vi "rsidr_core_global.vi"() -> ()   [LabVIEW 2020, in "Rohde&Schwarz RTx Oscilloscopes.lvlib"] (continued)
{"Level"=2, "Class Only"=TRUE, "Identifier"="", "Descriptive Name"="ARINC 429", "Data Type"=0, "Command"="", "Access"=0, "Range Table"="", "Read Callback"="", "Write Callback"="", "Supported Models"="", "Instrument Options"="", "Flags"=0, "Help"="ARINC 429 (Option K7)"}, {"Level"=3, "Class Only"=FALSE, "Identifier"="RSRTX_ATTR_PROTOCOL_ARINC429_SOURCE", "Descriptive Name"="Protocol ARINC429 Source", "Data Type"=0, "Command"="BUS{SerialBus}:ARINc:SOUR", "Access"=2, "Range Table"="rsrtx_rngSource", "Read Callback"="", "Write Callback"="", "Supported Models"="RTM|RTA", "Instrument Options"="", "Flags"=0, "Help"="Sets the channel for the signal source.\n\nAvailable Repeated Capabilities:\nSerialBus: SB1, SB2, SB3, SB4\r\n\nRemote-control command(s):\nBUS<b>:ARINc:SOURce"}, {"Level"=3, "Class Only"=FALSE, "Identifier"="RSRTX_ATTR_PROTOCOL_ARINC429_POLARITY", "Descriptive Name"="Protocol ARINC429 Polarity", "Data Type"=0, "Command"="BUS{SerialBus}:ARIN:POL", "Access"=2, "Range Table"="rsrtx_rngProtocolARINC429Polarity", "Read Callback"="", "Write Callback"="", "Supported Models"="RTM|RTA", "Instrument Options"="", "Flags"=0, "Help"="Sets the wire on which the bus signal is measured.\n\nAvailable Repeated Capabilities:\nSerialBus: SB1, SB2, SB3, SB4\r\n\nRemote-control command(s):\nBUS<b>:ARINc:POLarity"}, {"Level"=3, "Class Only"=FALSE, "Identifier"="RSRTX_ATTR_PROTOCOL_ARINC429_BIT_RATE_MODE", "Descriptive Name"="Protocol ARINC429 Bit Rate Mode", "Data Type"=0, "Command"="BUS{SerialBus}:ARIN:BRM", "Access"=2, "Range Table"="rsrtx_rngProtocolARINC429BitRateMode", "Read Callback"="", "Write Callback"="", "Supported Models"="RTM|RTA", "Instrument Options"="", "Flags"=0, "Help"="Sets the bit rate mode to high or low speed.\n\nAvailable Repeated Capabilities:\nSerialBus: SB1, SB2, SB3, SB4\r\n\nRemote-control command(s):\nBUS<b>:ARINc:BRMode"}, {"Level"=3, "Class Only"=FALSE, "Identifier"="RSRTX_ATTR_PROTOCOL_ARINC429_BIT_RATE", "Descriptive Name"="Protocol ARINC429 Bit Rate", "Data Type"=1, "Command"="BUS{SerialBus}:ARIN:BRV", "Access"=2, "Range Table"="", "Read Callback"="", "Write Callback"="", "Supported Models"="RTM|RTA", "Instrument Options"="", "Flags"=0, "Help"="Sets the number of transmitted bits per second.\n\nAvailable Repeated Capabilities:\nSerialBus: SB1, SB2, SB3, SB4\r\n\nRemote-control command(s):\nBUS<b>:ARINc:BRValue"}, {"Level"=3, "Class Only"=FALSE, "Identifier"="RSRTX_ATTR_PROTOCOL_ARINC429_THRESHOLD_HIGH", "Descriptive Name"="Protocol ARINC429 Threshold High", "Data Type"=1, "Command"="BUS{SerialBus}:ARIN:THR:HIGH", "Access"=2, "Range Table"="rsrtx_rngProtocolARINC429ThresholdHigh", "Read Callback"="", "Write Callback"="", "Supported Models"="RTM|RTA", "Instrument Options"="", "Flags"=0, "Help"="Sets the high threshold level of the signal.\n\nAvailable Repeated Capabilities:\nSerialBus: SB1, SB2, SB3, SB4\r\n\nRemote-control command(s):\nBUS<b>:ARINc:THReshold:HIGH"}, {"Level"=3, "Class Only"=FALSE, "Identifier"="RSRTX_ATTR_PROTOCOL_ARINC429_THRESHOLD_LOW", "Descriptive Name"="Protocol ARINC429 Threshold Low", "Data Type"=1, "Command"="BUS{SerialBus}:ARIN:THR:LOW", "Access"=2, "Range Table"="rsrtx_rngProtocolARINC429ThresholdLow", "Read Callback"="", "Write Callback"="", "Supported Models"="RTM|RTA", "Instrument Options"="", "Flags"=0, "Help"="Sets the low threshold level of the signal.\n\nAvailable Repeated Capabilities:\nSerialBus: SB1, SB2, SB3, SB4\r\n\nRemote-control command(s):\nBUS<b>:ARINc:THReshold:LOW"}, {"Level"=3, "Class Only"=FALSE, "Identifier"="RSRTX_ATTR_PROTOCOL_ARINC429_DATA_FORMAT", "Descriptive Name"="Protocol ARINC429 Data Format", "Data Type"=0, "Command"="BUS{SerialBus}:ARIN:DATA:FORM", "Access"=2, "Range Table"="rsrtx_rngProtocolARINC429DataFormat", "Read Callback"="", "Write Callback"="", "Supported Models"="RTM|RTA", "Instrument Options"="", "Flags"=0, "Help"="Sets the decoding data format for the specified ARINC 429 bus.\n\nAvailable Repeated Capabilities:\nSerialBus: SB1, SB2, SB3, SB4\r\n\nRemote-control command(s):\nBUS<b>:ARINc:DATA:FORMat"}, {"Level"=3, "Class Only"=TRUE, "Identifier"="", "Descriptive Name"="Decoding Results", "Data Type"=0, "Command"="", "Access"=0, "Range Table"="", "Read Callback"="", "Write Callback"="", "Supported Models"="", "Instrument Options"="", "Flags"=0, "Help"="Returns the decoding result of the specified word."}, {"Level"=4, "Class Only"=FALSE, "Identifier"="RSRTX_ATTR_PROTOCOL_ARINC429_WORD_COUNT", "Descriptive Name"="Protocol ARINC429 Word Count", "Data Type"=0, "Command"="BUS{SerialBus}:ARIN:WCO?", "Access"=0, "Range Table"="", "Read Callback"="", "Write Callback"="", "Supported Models"="RTM|RTA", "Instrument Options"="", "Flags"=0, "Help"="Returns the number of decoded words.\n\nAvailable Repeated Capabilities:\nSerialBus: SB1, SB2, SB3, SB4\r\n\nRemote-control command(s):\nBUS<b>:ARINc:WCOunt?"}, {"Level"=4, "Class Only"=FALSE, "Identifier"="RSRTX_ATTR_PROTOCOL_ARINC429_SELECTED_WORD", "Descriptive Name"="Protocol ARINC429 Selected Word", "Data Type"=0, "Command"="", "Access"=2, "Range Table"="", "Read Callback"="", "Write Callback"="", "Supported Models"="", "Instrument Options"="", "Flags"=0, "Help"="Sets selector repeated capability Word.\n\nAvailable Repeated Capabilities:\nNone\n\nRemote-control command(s):\n"}, {"Level"=4, "Class Only"=FALSE, "Identifier"="RSRTX_ATTR_PROTOCOL_ARINC429_WORD_STATUS", "Descriptive Name"="Protocol ARINC429 Word Status", "Data Type"=0, "Command"="BUS{SerialBus}:ARIN:WORD<Word>:STAT?", "Access"=0, "Range Table"="rsrtx_rngARINC429WordStatus", "Read Callback"="rsrtx_FormatARINCWordRepCapInt_ReadCallback.vi", "Write Callback"="", "Supported Models"="RTM|RTA", "Instrument Options"="", "Flags"=0, "Help"="Returns the status of the specified word.\n\nAvailable Repeated Capabilities:\nSerialBus: SB1, SB2, SB3, SB4\r\n\nRemote-control command(s):\nBUS<b>:ARINc:WORD<n>:STATus?"}, {"Level"=4, "Class Only"=FALSE, "Identifier"="RSRTX_ATTR_PROTOCOL_ARINC429_WORD_START", "Descriptive Name"="Protocol ARINC429 Word Start", "Data Type"=1, "Command"="BUS{SerialBus}:ARIN:WORD<Word>:STAR?", "Access"=0, "Range Table"="", "Read Callback"="rsrtx_FormatARINCWordRepCapReal_ReadCallback.vi", "Write Callback"="", "Supported Models"="RTM|RTA", "Instrument Options"="", "Flags"=0, "Help"="Returns the start time of the specified word.\n\nAvailable Repeated Capabilities:\nSerialBus: SB1, SB2, SB3, SB4\r\n\nRemote-control command(s):\nBUS<b>:ARINc:WORD<n>:STARt?"}, {"Level"=4, "Class Only"=FALSE, "Identifier"="RSRTX_ATTR_PROTOCOL_ARINC429_WORD_STOP", "Descriptive Name"="Protocol ARINC429 Word Stop", "Data Type"=1, "Command"="BUS{SerialBus}:ARIN:WORD<Word>:STOP?", "Access"=0, "Range Table"="", "Read Callback"="rsrtx_FormatARINCWordRepCapReal_ReadCallback.vi", "Write Callback"="", "Supported Models"="RTM|RTA", "Instrument Options"="", "Flags"=0, "Help"="Returns the start time of the specified word.\n\nAvailable Repeated Capabilities:\nSerialBus: SB1, SB2, SB3, SB4\r\n\nRemote-control command(s):\nBUS<b>:ARINc:WORD<n>:STOP?"}, {"Level"=4, "Class Only"=FALSE, "Identifier"="RSRTX_ATTR_PROTOCOL_ARINC429_WORD_SDI", "Descriptive Name"="Protocol ARINC429 Word SDI", "Data Type"=0, "Command"="BUS{SerialBus}:ARIN:WORD<Word>:SDI?", "Access"=0, "Range Table"="", "Read Callback"="rsrtx_FormatARINCWordRepCapInt_ReadCallback.vi", "Write Callback"="", "Supported Models"="RTM|RTA", "Instrument Options"="", "Flags"=0, "Help"="Returns the source/destination identifier (SDI) bits of the specified word.\n\nAvailable Repeated Capabilities:\nSerialBus: SB1, SB2, SB3, SB4\r\n\nRemote-control command(s):\nBUS<b>:ARINc:WORD<n>:SDI?"}, {"Level"=4, "Class Only"=FALSE, "Identifier"="RSRTX_ATTR_PROTOCOL_ARINC429_WORD_SSM", "Descriptive Name"="Protocol ARINC429 Word SSM", "Data Type"=0, "Command"="BUS{SerialBus}:ARIN:WORD<Word>:SSM?", "Access"=0, "Range Table"="", "Read Callback"="rsrtx_FormatARINCWordRepCapInt_ReadCallback.vi", "Write Callback"="", "Supported Models"="RTM|RTA", "Instrument Options"="", "Flags"=0, "Help"="Returns the source/destination identifier (SDI) bits of the specified word.\n\nAvailable Repeated Capabilities:\nSerialBus: SB1, SB2, SB3, SB4\r\n\nRemote-control command(s):\nBUS<b>:ARINc:WORD<n>:SSM?"}, {"Level"=4, "Class Only"=FALSE, "Identifier"="RSRTX_ATTR_PROTOCOL_ARINC429_WORD_LABEL", "Descriptive Name"="Protocol ARINC429 Word Label", "Data Type"=2, "Command"="BUS{SerialBus}:ARIN:WORD<Word>:LAB?", "Access"=0, "Range Table"="", "Read Callback"="rsrtx_FormatARINCWordRepCapString_ReadCallback.vi", "Write Callback"="", "Supported Models"="RTM|RTA", "Instrument Options"="", "Flags"=0, "Help"="Returns the label of the specified word.\n\nAvailable Repeated Capabilities:\nSerialBus: SB1, SB2, SB3, SB4\r\n\nRemote-control command(s):\nBUS<b>:ARINc:WORD<n>:LABel?"}, {"Level"=4, "Class Only"=FALSE, "Identifier"="RSRTX_ATTR_PROTOCOL_ARINC429_WORD_LABEL_VALUE", "Descriptive Name"="Protocol ARINC429 Word Label Value", "Data Type"=0, "Command"="BUS{SerialBus}:ARIN:WORD<Word>:LAB:VAL?", "Access"=0, "Range Table"="", "Read Callback"="rsrtx_FormatARINCWordRepCapInt_ReadCallback.vi", "Write Callback"="", "Supported Models"="RTM|RTA", "Instrument Options"="", "Flags"=0, "Help"="Returns the decimal value of the label of the specified word.\n\nAvailable Repeated Capabilities:\nSerialBus: SB1, SB2, SB3, SB4\r\n\nRemote-control command(s):\nBUS<b>:ARINc:WORD<n>:LABel[:VALue]?"}, {"Level"=4, "Class Only"=FALSE, "Identifier"="RSRTX_ATTR_PROTOCOL_ARINC429_WORD_PATTERN", "Descriptive Name"="Protocol ARINC429 Word Pattern", "Data Type"=0, "Command"="BUS{SerialBus}:ARIN:WORD<Word>:PATT?", "Access"=0, "Range Table"="", "Read Callback"="rsrtx_FormatARINCWordRepCapInt_ReadCallback.vi", "Write Callback"="", "Supported Models"="RTM|RTA", "Instrument Options"="", "Flags"=0, "Help"="Returns all 32 bits of a data word as decimal value.\n\nAvailable Repeated Capabilities:\nSerialBus: SB1, SB2, SB3, SB4\r\n\nRemote-control command(s):\nBUS<b>:ARINc:WORD<n>:PATTern?"}, {"Level"=4, "Class Only"=FALSE, "Identifier"="RSRTX_ATTR_PROTOCOL_ARINC429_WORD_PARITY", "Descriptive Name"="Protocol ARINC429 Word Parity", "Data Type"=0, "Command"="BUS{SerialBus}:ARIN:WORD<Word>:PAR?", "Access"=0, "Range Table"="", "Read Callback"="rsrtx_FormatARINCWordRepCapInt_ReadCallback.vi", "Write Callback"="", "Supported Models"="RTM|RTA", "Instrument Options"="", "Flags"=0, "Help"="Returns the parity of the specified word.\n\nAvailable Repeated Capabilities:\nSerialBus: SB1, SB2, SB3, SB4\r\n\nRemote-control command(s):\nBUS<b>:ARINc:WORD<n>:PARity?"}, {"Level"=4, "Class Only"=FALSE, "Identifier"="RSRTX_ATTR_PROTOCOL_ARINC429_WORD_FORMAT", "Descriptive Name"="Protocol ARINC429 Word Format", "Data Type"=0, "Command"="BUS{SerialBus}:ARIN:WORD<Word>:FORM?", "Access"=0, "Range Table"="rsrtx_rngProtocolARINC429DataFormat", "Read Callback"="rsrtx_FormatARINCWordRepCapInt_ReadCallback.vi", "Write Callback"="", "Supported Models"="RTM|RTA", "Instrument Options"="", "Flags"=0, "Help"="Returns the format of the sepcified word.\n\nAvailable Repeated Capabilities:\nSerialBus: SB1, SB2, SB3, SB4\r\n\nRemote-control command(s):\nBUS<b>:ARINc:WORD<n>:FORMat?"}, {"Level"=4, "Class Only"=FALSE, "Identifier"="RSRTX_ATTR_PROTOCOL_ARINC429_WORD_DATA", "Descriptive Name"="Protocol ARINC429 Word Data", "Data Type"=0, "Command"="BUS{SerialBus}:ARIN:WORD<Word>:DATA:VAL?", "Access"=0, "Range Table"="", "Read Callback"="rsrtx_FormatARINCWordRepCapInt_ReadCallback.vi", "Write Callback"="", "Supported Models"="", "Instrument Options"="", "Flags"=0, "Help"="Returns the decimal value of the data of the specified word.\n\nAvailable Repeated Capabilities:\nSerialBus: SB1, SB2, SB3, SB4\r\n\nRemote-control command(s):\nBUS<b>:ARINc:WORD<n>:DATA[:VALue]?"}, {"Level"=1, "Class Only"=TRUE, "Identifier"="", "Descriptive Name"="Power Analysis", "Data Type"=0, "Command"="", "Access"=0, "Range Table"="", "Read Callback"="", "Write Callback"="", "Supported Models"="", "Instrument Options"="", "Flags"=0, "Help"="Power Analysis."}, {"Level"=2, "Class Only"=FALSE, "Identifier"="RSRTX_ATTR_POWER_ANALYSIS_ENABLED", "Descriptive Name"="Power Analysis Enabled", "Data Type"=3, "Command"="POW:ENAB", "Access"=2, "Range Table"="", "Read Callback"="", "Write Callback"="", "Supported Models"="RTM|RTA", "Instrument Options"="", "Flags"=0, "Help"="Enables the power analysis.\n\nAvailable Repeated Capabilities:\nNone\n\nRemote-control command(s):\nPOWer:ENABle"}, {"Level"=2, "Class Only"=FALSE, "Identifier"="RSRTX_ATTR_POWER_ANALYSIS_TYPE", "Descriptive Name"="Power Analysis Type", "Data Type"=0, "Command"="POW:ATYP", "Access"=2, "Range Table"="rsrtx_rngPowerAnalysisType", "Read Callback"="", "Write Callback"="", "Supported Models"="RTM|RTA", "Instrument Options"="", "Flags"=0, "Help"="Selects power analysis type.\n\nAvailable Repeated Capabilities:\nNone\n\nRemote-control command(s):\nPOWer:ATYPe"}, {"Level"=2, "Class Only"=FALSE, "Identifier"="RSRTX_ATTR_POWER_ANALYSIS_RESULT_TABLE_ENABLED", "Descriptive Name"="Power Analysis Result Table Enabled", "Data Type"=3, "Command"="POW:RES:TABL", "Access"=2, "Range Table"="", "Read Callback"="", "Write Callback"="", "Supported Models"="RTM|RTA", "Instrument Options"="", "Flags"=0, "Help"="Displays or hides the result table. Available for harmonic and spectrum power measurements.\n\nAvailable Repeated Capabilities:\nNone\n\nRemote-control command(s):\nPOWer:RESult:TABLe"}, {"Level"=2, "Class Only"=FALSE, "Identifier"="RSRTX_ATTR_POWER_ANALYSIS_RESET_STATISTICS", "Descriptive Name"="Power Analysis Reset Statistics", "Data Type"=4, "Command"="POW:STAT:RES", "Access"=1, "Range Table"="", "Read Callback"="", "Write Callback"="", "Supported Models"="RTM|RTA", "Instrument Options"="", "Flags"=0, "Help"="Resets statistics.\n\nAvailable Repeated Capabilities:\nNone\n\nRemote-control command(s):\nPOWer:STATistics:RESet"}, {"Level"=2, "Class Only"=FALSE, "Identifier"="RSRTX_ATTR_POWER_ANALYSIS_STATISTICS_VISIBLE", "Descriptive Name"="Power Analysis Statistics Visible", "Data Type"=3, "Command"="POW:STAT:VIS", "Access"=2, "Range Table"="", "Read Callback"="", "Write Callback"="", "Supported Models"="RTM|RTA", "Instrument Options"="", "Flags"=0, "Help"="Visible statistics\n\nAvailable Repeated Capabilities:\nNone\n\nRemote-control command(s):\nPOWer:STATistics:VISible"}, {"Level"=2, "Class Only"=FALSE, "Identifier"="RSRTX_ATTR_POWER_ANALYSIS_START_DESKEW", "Descriptive Name"="Power Analysis Start Deskew", "Data Type"=4, "Command"="POW:DESK", "Access"=1, "Range Table"="", "Read Callback"="", "Write Callback"="", "Supported Models"="RTM|RTA", "Instrument Options"="", "Flags"=1, "Help"="Starts the automatic deskew procedure to align the waveforms of all visible channels. It is necessary to deskew if a current and a voltage probe is used in the measurment. Use the R&S RT-ZF20 power deskew fixture to deskew the probes.\n\nAvailable Repeated Capabilities:\nNone\n\nRemote-control command(s):\nPOWer:DESKew[:EXECute]"}, {"Level"=2, "Class Only"=FALSE, "Identifier"="RSRTX_ATTR_POWER_ANALYSIS_ZERO_OFFSET", "Descriptive Name"="Power Analysis Zero Offset", "Data Type"=4, "Command"="POW:ZOFF", "Access"=1, "Range Table"="", "Read Callback"="", "Write Callback"="", "Supported Models"="RTM|RTA", "Instrument Options"="", "Flags"=1, "Help"="Sets zero offset.\n\nAvailable Repeated Capabilities:\nNone\n\nRemote-control command(s):\nPOWer:ZOFFset[:EXECute]"}, {"Level"=2, "Class Only"=FALSE, "Identifier"="RSRTX_ATTR_POWER_ANALYSIS_AUTOSET", "Descriptive Name"="Power Analysis Autoset", "Data Type"=4, "Command"="POW:AUT", "Access"=1, "Range Table"="", "Read Callback"="", "Write Callback"="", "Supported Models"="RTM|RTA", "Instrument Options"="", "Flags"=0, "Help"="Starts power analysis autoset.\n\nAvailable Repeated Capabilities:\nNone\n\nRemote-control command(s):\nPOWer:AUToscale"}, {"Level"=2, "Class Only"=FALSE, "Identifier"="RSRTX_ATTR_POWER_ANALYSIS_AUTOSET_CURRENT", "Descriptive Name"="Power Analysis Autoset Current", "Data Type"=4, "Command"="POW:AUT:CURR", "Access"=1, "Range Table"="", "Read Callback"="", "Write Callback"="", "Supported Models"="RTM|RTA", "Instrument Options"="", "Flags"=0, "Help"="Starts power analysis current autoset.\n\nAvailable Repeated Capabilities:\nNone\n\nRemote-control command(s):\nPOWer:AUToscale:CURRent"}, {"Level"=2, "Class Only"=FALSE, "Identifier"="RSRTX_ATTR_POWER_ANALYSIS_AUTOSET_VOLTAGE", "Descriptive Name"="Power Analysis Autoset Voltage", "Data Type"=4, "Command"="POW:AUT:VOLT", "Access"=1, "Range Table"="", "Read Callback"="", "Write Callback"="", "Supported Models"="RTM|RTA", "Instrument Options"="", "Flags"=0, "Help"="Starts power analysis voltage autoset.\n\nAvailable Repeated Capabilities:\nNone\n\nRemote-control command(s):\nPOWer:AUToscale:VOLTage"}, {"Level"=2, "Class Only"=TRUE, "Identifier"="", "Descriptive Name"="Source", "Data Type"=0, "Command"="", "Access"=0, "Range Table"="", "Read Callback"="", "Write Callback"="", "Supported Models"="", "Instrument Options"="", "Flags"=0, "Help"="Clas for attributes with Source repcap."}, {"Level"=3, "Class Only"=FALSE, "Identifier"="RSRTX_ATTR_POWER_ANALYSIS_VOLTAGE_SOURCE", "Descriptive Name"="Power Analysis Voltage Source", "Data Type"=0, "Command"="POW:SOUR:VOLT{SourceNumber}", "Access"=2, "Range Table"="rsrtx_rngPowerAnalysisSource", "Read Callback"="", "Write Callback"="", "Supported Models"="RTM|RTA", "Instrument Options"="", "Flags"=0, "Help"="Sets the channel for the voltage source input.\n\nAvailable Repeated Capabilities:\nSourceNumber: S1, S2, S3, S4\r\n\nRemote-control command(s):\nPOWer:SOURce:VOLTage<n>"}, {"Level"=3, "Class Only"=FALSE, "Identifier"="RSRTX_ATTR_POWER_ANALYSIS_CURRENT_SOURCE", "Descriptive Name"="Power Analysis Current Source", "Data Type"=0, "Command"="POW:SOUR:CURR{SourceNumber}", "Access"=2, "Range Table"="rsrtx_rngPowerAnalysisSource", "Read Callback"="", "Write Callback"="", "Supported Models"="RTM|RTA", "Instrument Options"="", "Flags"=0, "Help"="Sets the channel for the current source input.\n\nAvailable Repeated Capabilities:\nSourceNumber: S1, S2, S3, S4\r\n\nRemote-control command(s):\nPOWer:SOURce:CURRent<n>"}, {"Level"=2, "Class Only"=TRUE, "Identifier"="", "Descriptive Name"="Report", "Data Type"=0, "Command"="", "Access"=0, "Range Table"="", "Read Callback"="", "Write Callback"="", "Supported Models"="", "Instrument Options"="", "Flags"=0, "Help"="Power analysis report."}, {"Level"=3, "Class Only"=FALSE, "Identifier"="RSRTX_ATTR_POWER_ANALYSIS_ADD_REPORT", "Descriptive Name"="Power Analysis Add Report", "Data Type"=4, "Command"="POW:REP:ADD", "Access"=1, "Range Table"="", "Read Callback"="", "Write Callback"="", "Supported Models"="RTM|RTA", "Instrument Options"="", "Flags"=0, "Help"="Adds a power report.\n\nAvailable Repeated Capabilities:\nNone\n\nRemote-control command(s):\nPOWer:REPort:ADD"}, {"Level"=3, "Class Only"=FALSE, "Identifier"="RSRTX_ATTR_POWER_ANALYSIS_REPORT_DUT", "Descriptive Name"="Power Analysis Report DUT", "Data Type"=2, "Command"="POW:REP:DUT", "Access"=2, "Range Table"="", "Read Callback"="", "Write Callback"="", "Supported Models"="RTM|RTA", "Instrument Options"="", "Flags"=0, "Help"="Sets a device under test (DUT) value that can be shown at the titel page of a report.\n\nAvailable Repeated Capabilities:\nNone\n\nRemote-control command(s):\nPOWer:REPort:DUT"}, {"Level"=3, "Class Only"=FALSE, "Identifier"="RSRTX_ATTR_POWER_ANALYSIS_REPORT_USER", "Descriptive Name"="Power Analysis Report User", "Data Type"=2, "Command"="POW:REP:USER", "Access"=2, "Range Table"="", "Read Callback"="", "Write Callback"="", "Supported Models"="RTM|RTA", "Instrument Options"="", "Flags"=0, "Help"="Sets a user value that can be shown at the titel page of a report.\n\nAvailable Repeated Capabilities:\nNone\n\nRemote-control command(s):\nPOWer:REPort:USER"}, {"Level"=3, "Class Only"=FALSE, "Identifier"="RSRTX_ATTR_POWER_ANALYSIS_REPORT_SITE", "Descriptive Name"="Power Analysis Report Site", "Data Type"=2, "Command"="POW:REP:SITE", "Access"=2, "Range Table"="", "Read Callback"="", "Write Callback"="", "Supported Models"="RTM|RTA", "Instrument Options"="", "Flags"=0, "Help"="Sets a site value that can be shown at the titel page of a report.\n\nAvailable Repeated Capabilities:\nNone\n\nRemote-control command(s):\nPOWer:REPort:SITE"}, {"Level"=3, "Class Only"=FALSE, "Identifier"="RSRTX_ATTR_POWER_ANALYSIS_REPORT_TEMPERATURE", "Descriptive Name"="Power Analysis Report Temperature", "Data Type"=0, "Command"="POW:REP:TEMP", "Access"=2, "Range Table"="rsrtx_rngPowerAnalysisReportTemperature", "Read Callback"="", "Write Callback"="", "Supported Models"="RTM|RTA", "Instrument Options"="", "Flags"=0, "Help"="Sets a temperature value that can be shown at the titel page of a report.\n\nAvailable Repeated Capabilities:\nNone\n\nRemote-control command(s):\nPOWer:REPort:TEMPerature"}, {"Level"=3, "Class Only"=FALSE, "Identifier"="RSRTX_ATTR_POWER_ANALYSIS_REPORT_DESCRIPTION", "Descriptive Name"="Power Analysis Report Description", "Data Type"=2, "Command"="POW:REP:DESC", "Access"=2, "Range Table"="", "Read Callback"="", "Write Callback"="", "Supported Models"="RTM|RTA", "Instrument Options"="", "Flags"=0, "Help"="Sets a description that can be shown at the titel page of a report.\n\nAvailable Repeated Capabilities:\nNone\n\nRemote-control command(s):\nPOWer:REPort:DESCription"}, {"Level"=3, "Class Only"=FALSE, "Identifier"="RSRTX_ATTR_POWER_ANALYSIS_REPORT_OUTPUT_FOLDER", "Descriptive Name"="Power Analysis Report Output Folder", "Data Type"=2, "Command"="POW:REP:OUTP", "Access"=2, "Range Table"="", "Read Callback"="", "Write Callback"="", "Supported Models"="RTM|RTA", "Instrument Options"="", "Flags"=0, "Help"="Sets the directory for the output folder, where the reports are stored.\n\nAvailable Repeated Capabilities:\nNone\n\nRemote-control command(s):\nPOWer:REPort:OUTPut"}, {"Level"=2, "Class Only"=TRUE, "Identifier"="", "Descriptive Name"="Power Quality Measurement", "Data Type"=0, "Command"="", "Access"=0, "Range Table"="", "Read Callback"="", "Write Callback"="", "Supported Models"="", "Instrument Options"="", "Flags"=0, "Help"="The &quot;Power Quality&quot; analysis measurements include the real power, the reactive power and the apparent power as well as the power factor. The crest factors and the phase angle between the current and voltage are also measured. These properties describe the power transfer in the system and allow you to characterize the power quality of the system."}, {"Level"=3, "Class Only"=FALSE, "Identifier"="RSRTX_ATTR_START_POWER_QUALITY_MEASUREMENT", "Descriptive Name"="Start Power Quality Measurement", "Data Type"=4, "Command"="POW:QUAL:EXEC", "Access"=1, "Range Table"="", "Read Callback"="", "Write Callback"="", "Supported Models"="RTM|RTA", "Instrument Options"="", "Flags"=0, "Help"="Starts the power quality measurement.\n\nAvailable Repeated Capabilities:\nNone\n\nRemote-control command(s):\nPOWer:QUALity:EXECute"}, {"Level"=3, "Class Only"=FALSE, "Identifier"="RSRTX_ATTR_POWER_QUALITY_MEASUREMENT_ADD_REPORT", "Descriptive Name"="Power Quality Measurement Add Report", "Data Type"=4, "Command"="POW:QUAL:REP:ADD", "Access"=1, "Range Table"="", "Read Callback"="", "Write Callback"="", "Supported Models"="RTM|RTA", "Instrument Options"="", "Flags"=1, "Help"="Adds the result to the report list.\n\nAvailable Repeated Capabilities:\nNone\n\nRemote-control command(s):\nPOWer:QUALity:REPort:ADD"}, {"Level"=3, "Class Only"=TRUE, "Identifier"="", "Descriptive Name"="Results", "Data Type"=0, "Command"="", "Access"=0, "Range Table"="", "Read Callback"="", "Write Callback"="", "Supported Models"="", "Instrument Options"="", "Flags"=0, "Help"="Power quality measurement results."}, {"Level"=2, "Class Only"=TRUE, "Identifier"="", "Descriptive Name"="Consumption Measurement", "Data Type"=0, "Command"="", "Access"=0, "Range Table"="", "Read Callback"="", "Write Callback"="", "Supported Models"="", "Instrument Options"="", "Flags"=0, "Help"="Consumption Measurement."}, {"Level"=3, "Class Only"=FALSE, "Identifier"="RSRTX_ATTR_START_POWER_CONSUMPTION_MEASUREMENT", "Descriptive Name"="Start Power Consumption Measurement", "Data Type"=4, "Command"="POW:CONS:EXEC", "Access"=1, "Range Table"="", "Read Callback"="", "Write Callback"="", "Supported Models"="RTM|RTA", "Instrument Options"="", "Flags"=0, "Help"="Start power consumption measurement.\n\nAvailable Repeated Capabilities:\nNone\n\nRemote-control command(s):\nPOWer:CONSumption:EXECute"}, {"Level"=3, "Class Only"=FALSE, "Identifier"="RSRTX_ATTR_RESTART_POWER_CONSUMPTION_MEASUREMENT", "Descriptive Name"="Restart Power Consumption Measurement", "Data Type"=4, "Command"="POW:CONS:REST", "Access"=1, "Range Table"="", "Read Callback"="", "Write Callback"="", "Supported Models"="RTM|RTA", "Instrument Options"="", "Flags"=0, "Help"="Restart power consumption measurement.\n\nAvailable Repeated Capabilities:\nNone\n\nRemote-control command(s):\nPOWer:CONSumption:RESTart"}, {"Level"=3, "Class Only"=FALSE, "Identifier"="RSRTX_ATTR_POWER_CONSUMPTION_MEASUREMENT_ADD_REPORT", "Descriptive Name"="Power Consumption Measurement Add Report", "Data Type"=4, "Command"="POW:CONS:REP:ADD", "Access"=1, "Range Table"="", "Read Callback"="", "Write Callback"="", "Supported Models"="RTM|RTA", "Instrument Options"="", "Flags"=1, "Help"="Adds the result to the report list.\n\nAvailable Repeated Capabilities:\nNone\n\nRemote-control command(s):\nPOWer:CONSumption:REPort:ADD"}, {"Level"=3, "Class Only"=TRUE, "Identifier"="", "Descriptive Name"="Results", "Data Type"=0, "Command"="", "Access"=0, "Range Table"="", "Read Callback"="", "Write Callback"="", "Supported Models"="", "Instrument Options"="", "Flags"=0, "Help"="Power consumption measurement results."}, {"Level"=4, "Class Only"=FALSE, "Identifier"="RSRTX_ATTR_POWER_CONSUMPTION_MEASUREMENT_DURATION_RESULT", "Descriptive Name"="Power Consumption Measurement Duration Result", "Data Type"=1, "Command"="POW:CONS:RES:DUR?", "Access"=0, "Range Table"="", "Read Callback"="", "Write Callback"="", "Supported Models"="RTM|RTA", "Instrument Options"="", "Flags"=0, "Help"="Returns the result of the measurement.\n\nAvailable Repeated Capabilities:\nNone\n\nRemote-control command(s):\nPOWer:CONSumption:RESult:DURation?"}, {"Level"=4, "Class Only"=FALSE, "Identifier"="RSRTX_ATTR_POWER_CONSUMPTION_MEASUREMENT_ENERGY_RESULT", "Descriptive Name"="Power Consumption Measurement Energy Result", "Data Type"=1, "Command"="POW:CONS:RES:ENER?", "Access"=0, "Range Table"="", "Read Callback"="", "Write Callback"="", "Supported Models"="RTM|RTA", "Instrument Options"="", "Flags"=0, "Help"="Returns the result of the measurement.\n\nAvailable Repeated Capabilities:\nNone\n\nRemote-control command(s):\nPOWer:CONSumption:RESult:ENERgy?"}, {"Level"=4, "Class Only"=FALSE, "Identifier"="RSRTX_ATTR_POWER_CONSUMPTION_MEASUREMENT_ACTIVE_RESULT", "Descriptive Name"="Power Consumption Measurement Active Result", "Data Type"=1, "Command"="POW:CONS:RES:REAL?", "Access"=0, "Range Table"="", "Read Callback"="", "Write Callback"="", "Supported Models"="RTM|RTA", "Instrument Options"="", "Flags"=0, "Help"="Returns the result of the measurement.\n\nAvailable Repeated Capabilities:\nNone\n\nRemote-control command(s):\nPOWer:CONSumption:RESult:REALpower?"}, {"Level"=4, "Class Only"=FALSE, "Identifier"="RSRTX_ATTR_POWER_CONSUMPTION_MEASUREMENT_APPARENT_POWER_RESULT", "Descriptive Name"="Power Consumption Measurement Apparent Power Result", "Data Type"=1, "Command"="POW:CONS:RES:APP?", "Access"=0, "Range Table"="", "Read Callback"="", "Write Callback"="", "Supported Models"="RTM|RTA", "Instrument Options"="", "Flags"=0, "Help"="Returns the Apparent Power result of the measurement.\n\nAvailable Repeated Capabilities:\nNone\n\nRemote-control command(s):\nPOWer:CONSumption:RESult:APParent?"}, {"Level"=4, "Class Only"=FALSE, "Identifier"="RSRTX_ATTR_POWER_CONSUMPTION_MEASUREMENT_POWER_FACTOR_RESULT", "Descriptive Name"="Power Consumption Measurement Power Factor Result", "Data Type"=1, "Command"="POW:CONS:RES:PFAC?", "Access"=0, "Range Table"="", "Read Callback"="", "Write Callback"="", "Supported Models"="RTM|RTA", "Instrument Options"="", "Flags"=0, "Help"="Returns the Power Factor result of the measurement.\n\nAvailable Repeated Capabilities:\nNone\n\nRemote-control command(s):\nPOWer:CONSumption:RESult:PFACtor?"}, {"Level"=4, "Class Only"=FALSE, "Identifier"="RSRTX_ATTR_POWER_CONSUMPTION_MEASUREMENT_PHASE_RESULT", "Descriptive Name"="Power Consumption Measurement Phase Result", "Data Type"=1, "Command"="POW:CONS:RES:PHAS?", "Access"=0, "Range Table"="", "Read Callback"="", "Write Callback"="", "Supported Models"="RTM|RTA", "Instrument Options"="", "Flags"=0, "Help"="Returns the phase result of the measurement.\n\nAvailable Repeated Capabilities:\nNone\n\nRemote-control command(s):\nPOWer:CONSumption:RESult:PHASe?"}, {"Level"=4, "Class Only"=FALSE, "Identifier"="RSRTX_ATTR_POWER_CONSUMPTION_MEASUREMENT_REACTIVE_POWER_RESULT", "Descriptive Name"="Power Consumption Measurement Reactive Power Result", "Data Type"=1, "Command"="POW:CONS:RES:REAC?", "Access"=0, "Range Table"="", "Read Callback"="", "Write Callback"="", "Supported Models"="RTM|RTA", "Instrument Options"="", "Flags"=0, "Help"="Returns the Reactive Power result of the measurement.\n\nAvailable Repeated Capabilities:\nNone\n\nRemote-control command(s):\nPOWer:CONSumption:RESult:REACtive?"}, {"Level"=2, "Class Only"=TRUE, "Identifier"="", "Descriptive Name"="Current Harmonics Measurement", "Data Type"=0, "Command"="", "Access"=0, "Range Table"="", "Read Callback"="", "Write Callback"="", "Supported Models"="", "Instrument Options"="", "Flags"=0, "Help"="Current Harmonics Measurement."}, {"Level"=3, "Class Only"=FALSE, "Identifier"="RSRTX_ATTR_START_POWER_CURRENT_HARMONICS_MEASUREMENT", "Descriptive Name"="Start Power Current Harmonics Measurement", "Data Type"=4, "Command"="POW:HARM:EXEC", "Access"=1, "Range Table"="", "Read Callback"="", "Write Callback"="", "Supported Models"="RTM|RTA", "Instrument Options"="", "Flags"=1, "Help"="Start power current harmonics measurement.\n\nAvailable Repeated Capabilities:\nNone\n\nRemote-control command(s):\nPOWer:HARMonics:EXECute"}, {"Level"=3, "Class Only"=FALSE, "Identifier"="RSRTX_ATTR_POWER_CURRENT_HARMONICS_MEASUREMENT_STANDARD", "Descriptive Name"="Power Current Harmonics Measurement Standard", "Data Type"=0, "Command"="POW:HARM:STAN", "Access"=2, "Range Table"="rsrtx_rngHarmonicsStandard", "Read Callback"="", "Write Callback"="", "Supported Models"="RTM|RTA", "Instrument Options"="", "Flags"=0, "Help"="Selects current harmonics standard.\n\nAvailable Repeated Capabilities:\nNone\n\nRemote-control command(s):\nPOWer:HARMonics:STANdard"}, {"Level"=3, "Class Only"=FALSE, "Identifier"="RSRTX_ATTR_POWER_CURRENT_HARMONICS_MEASUREMENT_FUNDAMENTAL", "Descriptive Name"="Power Current Harmonics Measurement Fundamental", "Data Type"=0, "Command"="POW:HARM:ENFR", "Access"=2, "Range Table"="rsrtx_rngHarmonicsFundamental", "Read Callback"="", "Write Callback"="", "Supported Models"="RTM|RTA", "Instrument Options"="", "Flags"=0, "Help"="Configures current harmonics fundamental.\n\nAvailable Repeated Capabilities:\nNone\n\nRemote-control command(s):\nPOWer:HARMonics:ENFRequency"}, {"Level"=3, "Class Only"=FALSE, "Identifier"="RSRTX_ATTR_POWER_CURRENT_HARMONICS_MEASUREMENT_FUNDAMENTAL_MIL", "Descriptive Name"="Power Current Harmonics Measurement Fundamental MIL", "Data Type"=0, "Command"="POW:HARM:MIFR", "Access"=2, "Range Table"="rsrtx_rngHarmonicsFundamentalMIL", "Read Callback"="", "Write Callback"="", "Supported Models"="RTM|RTA", "Instrument Options"="", "Flags"=0, "Help"="Selects the frequency of the input signal when Standard is set to MIL.\n\nAvailable Repeated Capabilities:\nNone\n\nRemote-control command(s):\nPOWer:HARMonics:MIFRequency"}, {"Level"=3, "Class Only"=FALSE, "Identifier"="RSRTX_ATTR_POWER_CURRENT_HARMONICS_MEASUREMENT_FUNDAMENTAL_RTC", "Descriptive Name"="Power Current Harmonics Measurement Fundamental RTC", "Data Type"=0, "Command"="POW:HARM:DOFR", "Access"=2, "Range Table"="rsrtx_rngHarmonicsFundamentalRTC", "Read Callback"="", "Write Callback"="", "Supported Models"="RTM|RTA", "Instrument Options"="", "Flags"=0, "Help"="Selects the frequency of the input signal when Standard is set to RTC.\n\nAvailable Repeated Capabilities:\nNone\n\nRemote-control command(s):\nPOWer:HARMonics:DOFRequency"}, {"Level"=3, "Class Only"=FALSE, "Identifier"="RSRTX_ATTR_POWER_CURRENT_HARMONICS_NUMBER_OF_MEASURED_HARMONICS", "Descriptive Name"="Power Current Harmonics Number Of Measured Harmonics", "Data Type"=0, "Command"="POW:HARM:AVA?", "Access"=0, "Range Table"="", "Read Callback"="", "Write Callback"="", "Supported Models"="RTM|RTA", "Instrument Options"="", "Flags"=0, "Help"="Returns the number of measured harmonics.\n\nAvailable Repeated Capabilities:\nNone\n\nRemote-control command(s):\nPOWer:HARMonics:AVAilable?"}, {"Level"=3, "Class Only"=FALSE, "Identifier"="RSRTX_ATTR_POWER_CURRENT_HARMONICS_MEASUREMENT_ADD_REPORT", "Descriptive Name"="Power Current Harmonics Measurement Add Report", "Data Type"=4, "Command"="POW:HARM:REP:ADD", "Access"=1, "Range Table"="", "Read Callback"="", "Write Callback"="", "Supported Models"="RTM|RTA", "Instrument Options"="", "Flags"=1, "Help"="Adds the result to the report list.\n\nAvailable Repeated Capabilities:\nNone\n\nRemote-control command(s):\nPOWer:HARMonics:REPort:ADD"}, {"Level"=3, "Class Only"=FALSE, "Identifier"="RSRTX_ATTR_POWER_CURRENT_HARMONICS_MEASUREMENT_DURATION", "Descriptive Name"="Power Current Harmonics Measurement Duration", "Data Type"=1, "Command"="POW:HARM:MEAS:DUR?", "Access"=0, "Range Table"="", "Read Callback"="", "Write Callback"="", "Supported Models"="RTM|RTA", "Instrument Options"="", "Flags"=0, "Help"="Returns the measurement duration.\n\nAvailable Repeated Capabilities:\nNone\n\nRemote-control command(s):\nPOWer:HARMonics:MEASurement:DURation?"}, {"Level"=3, "Class Only"=TRUE, "Identifier"="", "Descriptive Name"="Results", "Data Type"=0, "Command"="", "Access"=0, "Range Table"="", "Read Callback"="", "Write Callback"="", "Supported Models"="", "Instrument Options"="", "Flags"=0, "Help"="Current harmonics measurement results."}, {"Level"=4, "Class Only"=FALSE, "Identifier"="RSRTX_ATTR_POWER_CURRENT_HARMONICS_MEASUREMENT_LIMIT_CHECK_RESULT", "Descriptive Name"="Power Current Harmonics Measurement Limit Check Result", "Data Type"=0, "Command"="POW:HARM:RES{ResultNumber}:VAL?", "Access"=0, "Range Table"="rsrtx_rngLimitCheck", "Read Callback"="", "Write Callback"="", "Supported Models"="RTM|RTA", "Instrument Options"="", "Flags"=0, "Help"="Returns the limit check result.\n\nAvailable Repeated Capabilities:\nResultNumber: Res1, Res2, Res3, Res4, Res5, Res6, Res7, Res8, Res9, Res10, Res11, Res12, Res13, Res14, Res15, Res16, Res17, Res18, Res19, Res20, Res21, Res22, Res23, Res24, Res25, Res26, Res27, Res28, Res29, Res30, Res31, Res32, Res33, Res34, Res35, Res36, Res37, Res38, Res39, Res40\r\n\nRemote-control command(s):\nPOWer:HARMonics:RESult<n>:VALid?"}, {"Level"=4, "Class Only"=FALSE, "Identifier"="RSRTX_ATTR_RESET_POWER_CURRENT_HARMONICS_MEASUREMENT_RESULTS", "Descriptive Name"="Reset Power Current Harmonics Measurement Results", "Data Type"=4, "Command"="POW:HARM:RES{ResultNumber}:RES", "Access"=1, "Range Table"="", "Read Callback"="", "Write Callback"="", "Supported Models"="RTM|RTA", "Instrument Options"="", "Flags"=0, "Help"="Resets the results.\n\nAvailable Repeated Capabilities:\nResultNumber: Res1, Res2, Res3, Res4, Res5, Res6, Res7, Res8, Res9, Res10, Res11, Res12, Res13, Res14, Res15, Res16, Res17, Res18, Res19, Res20, Res21, Res22, Res23, Res24, Res25, Res26, Res27, Res28, Res29, Res30, Res31, Res32, Res33, Res34, Res35, Res36, Res37, Res38, Res39, Res40\r\n\nRemote-control command(s):\nPOWer:HARMonics:RESult<n>:RESet"}, {"Level"=3, "Class Only"=TRUE, "Identifier"="", "Descriptive Name"="Frequency Results", "Data Type"=0, "Command"="", "Access"=0, "Range Table"="", "Read Callback"="", "Write Callback"="", "Supported Models"="", "Instrument Options"="", "Flags"=0, "Help"="Current harmonics measurement frequency results."}, {"Level"=4, "Class Only"=FALSE, "Identifier"="RSRTX_ATTR_POWER_CURRENT_HARMONICS_MEASUREMENT_FREQUENCY_CURRENT", "Descriptive Name"="Power Current Harmonics Measurement Frequency Current", "Data Type"=1, "Command"="POW:HARM:MEAS:FREQ?", "Access"=0, "Range Table"="", "Read Callback"="", "Write Callback"="", "Supported Models"="RTM|RTA", "Instrument Options"="", "Flags"=0, "Help"="Returns the current frequency value.\n\nAvailable Repeated Capabilities:\nNone\n\nRemote-control command(s):\nPOWer:HARMonics:MEASurement:FREQuency[:ACTual]?"}, {"Level"=4, "Class Only"=FALSE, "Identifier"="RSRTX_ATTR_POWER_CURRENT_HARMONICS_MEASUREMENT_FREQUENCY_AVERAGE", "Descriptive Name"="Power Current Harmonics Measurement Frequency Average", "Data Type"=1, "Command"="POW:HARM:MEAS:FREQ:AVG?", "Access"=0, "Range Table"="", "Read Callback"="", "Write Callback"="", "Supported Models"="RTM|RTA", "Instrument Options"="", "Flags"=0, "Help"="Returns the average frequency of the measured signal.\n\nAvailable Repeated Capabilities:\nNone\n\nRemote-control command(s):\nPOWer:HARMonics:MEASurement:FREQuency:AVG?"}, {"Level"=4, "Class Only"=FALSE, "Identifier"="RSRTX_ATTR_POWER_CURRENT_HARMONICS_MEASUREMENT_FREQUENCY_MAXIMUM", "Descriptive Name"="Power Current Harmonics Measurement Frequency Maximum", "Data Type"=1, "Command"="POW:HARM:MEAS:FREQ:PPE?", "Access"=0, "Range Table"="", "Read Callback"="", "Write Callback"="", "Supported Models"="RTM|RTA", "Instrument Options"="", "Flags"=0, "Help"="Returns the maximum frequency of the measured signal.\n\nAvailable Repeated Capabilities:\nNone\n\nRemote-control command(s):\nPOWer:HARMonics:MEASurement:FREQuency:PPEak?"}, {"Level"=4, "Class Only"=FALSE, "Identifier"="RSRTX_ATTR_POWER_CURRENT_HARMONICS_MEASUREMENT_FREQUENCY_MINIMUM", "Descriptive Name"="Power Current Harmonics Measurement Frequency Minimum", "Data Type"=1, "Command"="POW:HARM:MEAS:FREQ:NPE?", "Access"=0, "Range Table"="", "Read Callback"="", "Write Callback"="", "Supported Models"="RTM|RTA", "Instrument Options"="", "Flags"=0, "Help"="Returns the minimum frequency of the measured signal.\n\nAvailable Repeated Capabilities:\nNone\n\nRemote-control command(s):\nPOWer:HARMonics:MEASurement:FREQuency:NPEak?"}, {"Level"=4, "Class Only"=FALSE, "Identifier"="RSRTX_ATTR_POWER_CURRENT_HARMONICS_MEASUREMENT_FREQUENCY_STANDARD_DEVIATION", "Descriptive Name"="Power Current Harmonics Measurement Frequency Standard Deviation", "Data Type"=1, "Command"="POW:HARM:MEAS:FREQ:STDD?", "Access"=0, "Range Table"="", "Read Callback"="", "Write Callback"="", "Supported Models"="RTM|RTA", "Instrument Options"="", "Flags"=0, "Help"="Returns the standard deviation of frequencies of the measured signal.\n\nAvailable Repeated Capabilities:\nNone\n\nRemote-control command(s):\nPOWer:HARMonics:MEASurement:FREQuency:STDDev?"}, {"Level"=3, "Class Only"=TRUE, "Identifier"="", "Descriptive Name"="Real Power Results", "Data Type"=0, "Command"="", "Access"=0, "Range Table"="", "Read Callback"="", "Write Callback"="", "Supported Models"="", "Instrument Options"="", "Flags"=0, "Help"="Current harmonics measurement real power results."}, {"Level"=4, "Class Only"=FALSE, "Identifier"="RSRTX_ATTR_POWER_CURRENT_HARMONICS_MEASUREMENT_REAL_POWER_CURRENT", "Descriptive Name"="Power Current Harmonics Measurement Real Power Current", "Data Type"=1, "Command"="POW:HARM:MEAS:REAL?", "Access"=0, "Range Table"="", "Read Callback"="", "Write Callback"="", "Supported Models"="RTM|RTA", "Instrument Options"="", "Flags"=0, "Help"="Returns the current real power value.\n\nAvailable Repeated Capabilities:\nNone\n\nRemote-control command(s):\nPOWer:HARMonics:MEASurement:REALpower[:ACTual]?"}, {"Level"=3, "Class Only"=TRUE, "Identifier"="", "Descriptive Name"="Total Harmonic Distortion Results", 
